vi "State Machine.vi"() -> ()   [LabVIEW 2013]
uses:
  StateEnum.ctl
panel:
  in  "Menu":T1
  # "You must also the order in\nthis cluster"
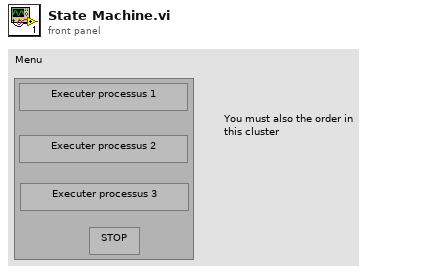
[diagram p1: front panel]
types:
  T1 = cluster{"Executer processus 1":bool, bool, bool, "STOP":bool}
  T2 = typedef "StateEnum.ctl" = enum32{"Inactif", "Processus 1", "Processus 2", "Processus 3", "Arret"}
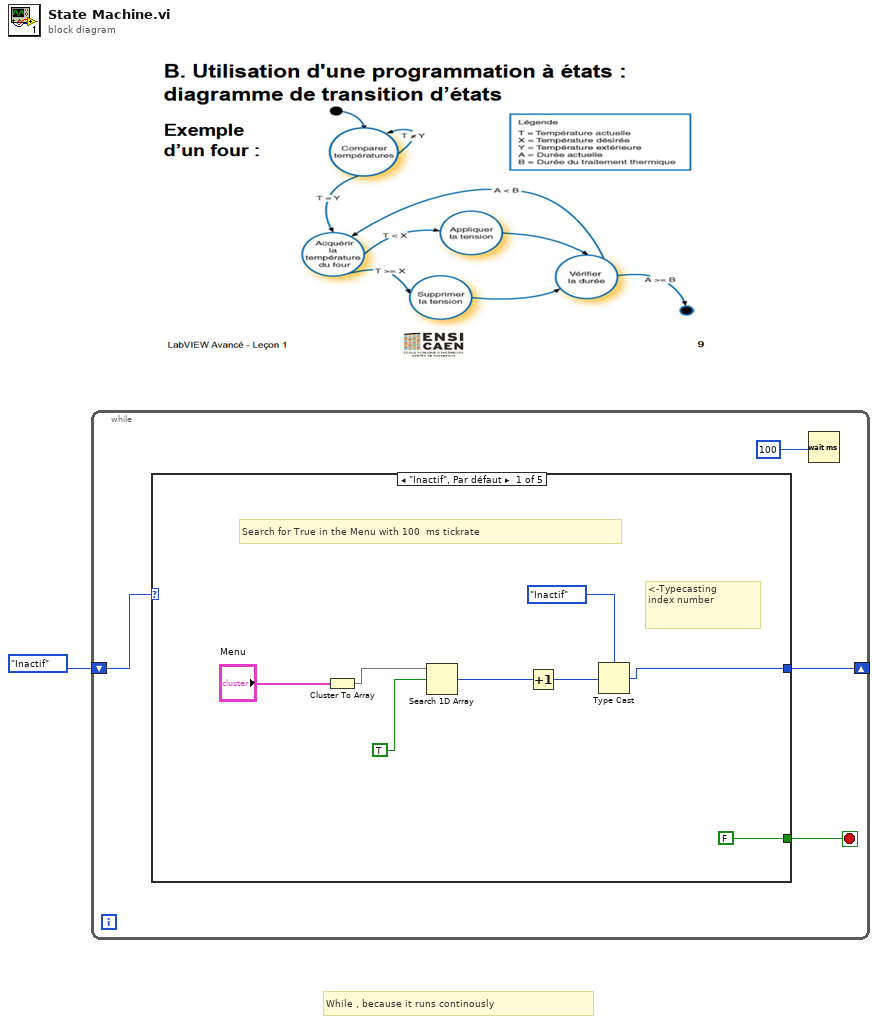
[diagram p0: block diagram]
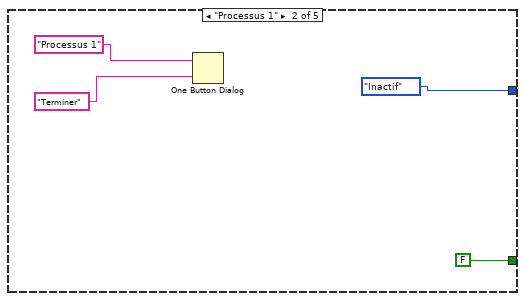
[diagram p2: hidden frame]
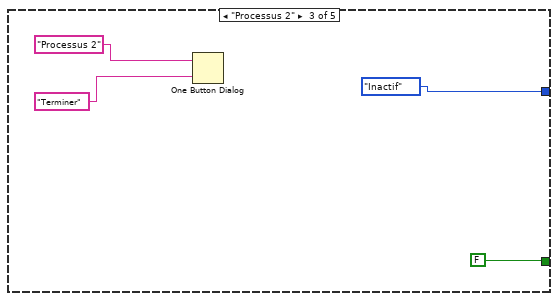
[diagram p3: hidden frame]
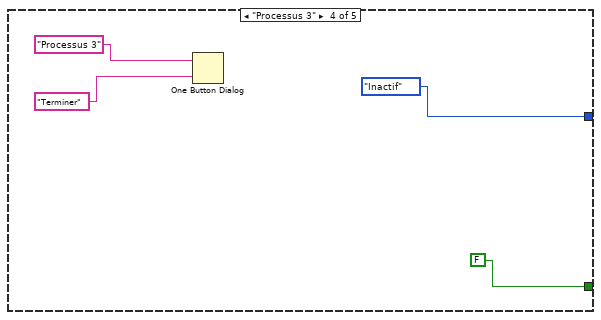
[diagram p4: hidden frame]
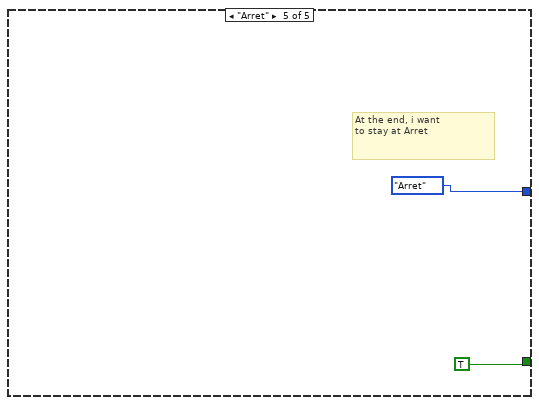
[diagram p5: hidden frame]
diagram:
  # "While , because it runs continously"
  n1 = while {
    shift-right: [w3] -> _
    shift-left: StateEnum."Inactif" ("Énum d'etats") -> [w5]
    stop <- w4 stop-if-true
    n2 = case shown="\"Inactif\", Par défaut" w5 {
      tunnel: [FALSE FALSE FALSE FALSE TRUE] -> w4
      tunnel: [w6 StateEnum."Inactif" ("Énum d'etats") StateEnum."Inactif" ("Énum d'etats") StateEnum."Inactif" ("Énum d'etats") StateEnum."Arret" ("Énum d'etats")] -> w3
      frame "Inactif", Default {
        # "<-Typecasting\nindex number"
        # "Search for True in the Menu with 100  ms tickrate"
        n3 = Cluster To Array(cluster="Menu") -> (array=w13:bool[])
        n4 = Search 1D Array(1D array=w13, element=TRUE) -> (index of element=w9:i32)  [unwired: 1 in]
        n5 = Increment(x=w9) -> (x+1=w8:i32)
        n6 = Type Cast(type=StateEnum."Inactif" ("Énum d'etats"), x=w8) -> (*(type *) &x=w6:T2)
      }
      frame "Processus 1" {
        n7 = One Button Dialog(message="Processus 1", button name ("OK")="Terminer") -> ()  [unwired: 1 out]
      }
      frame "Processus 2" {
        n8 = One Button Dialog(message="Processus 2", button name ("OK")="Terminer") -> ()  [unwired: 1 out]
      }
      frame "Processus 3" {
        n9 = One Button Dialog(message="Processus 3", button name ("OK")="Terminer") -> ()  [unwired: 1 out]
      }
      frame "Arret" {
        # "At the end, i want\nto stay at Arret"
      }
    }
    n10 = Wait (ms)(milliseconds to wait=100) -> ()  [unwired: 1 out]
  }
